vi "Update Routing Channel Name.vi"(8 "error in (no error)":errorcluster, 10 "New Channel Name":string, 11 "Channel Ref in":T1 format="%.0x") -> (0 "error out":errorcluster, 3 "Channel Ref out":T1 format="%.0x")   [LabVIEW 2017, in "SLSC Switch Scripting.lvlib"]
uses:
  SLSC Switch Scripting.lvlib
  <vilib>/NI Veristand/Custom Device API/Custom Device Item Ref.ctl
  <vilib>/NI VeriStand/Custom Device API/Custom Device API.lvlib
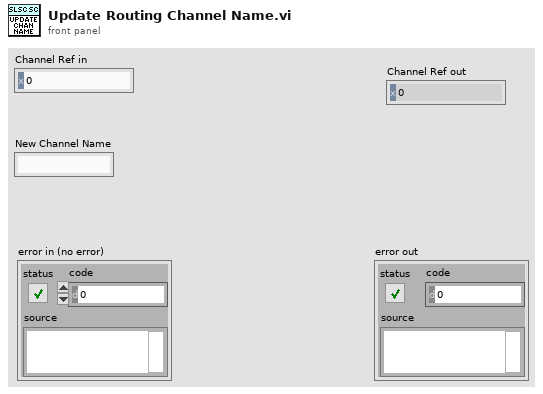
[diagram p1: front panel]
types:
  T1 = typedef "Custom Device API.lvlib/Custom Device Item Ref.ctl" = u64
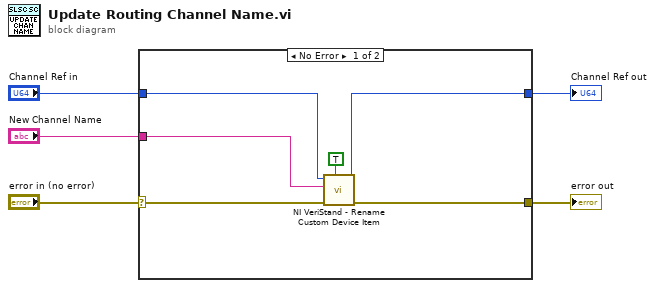
[diagram p0: block diagram]
diagram:
  n1 = case shown="No Error" "error in (no error)" {
    selector: "error in (no error)" -> [w7 w13]
    tunnel: [w9 w13] -> w5
    tunnel: [w10 w12] -> w4
    tunnel: "Channel Ref in" -> [w11 w12]
    tunnel: "New Channel Name" -> [w8 _]
    frame No Error {
      n2 = call <vilib>:"NI VeriStand - Rename Custom Device Item.vi"("Force Rename (F)"=TRUE, "error in (no error)"=w7, "New Name"=w8, "Item Ref in"=w11) -> ("error out"=w9:errorcluster, "Item Ref out"=w10:T1)  [unwired: 5 in, 1 out]
    }
    frame Error {
    }
  }
  "error out" <- w5
  "Channel Ref out" <- w4
